vi "Get Response Fit.vi"(8 "error in (no error)":errorcluster, 11 "Exponential Fit in":refnum<class "Exponential Fit.lvclass">) -> (0 "error out":errorcluster, 2 "Fit out":dbl[](array[numeric]), 3 "Exponential Fit out":refnum<class "Exponential Fit.lvclass">)   [LabVIEW 2016, in "Exponential Fit.lvclass"]
uses:
  Exponential Fit.lvclass
  Exponential Fit.lvclass/Exponential Fit.ctl
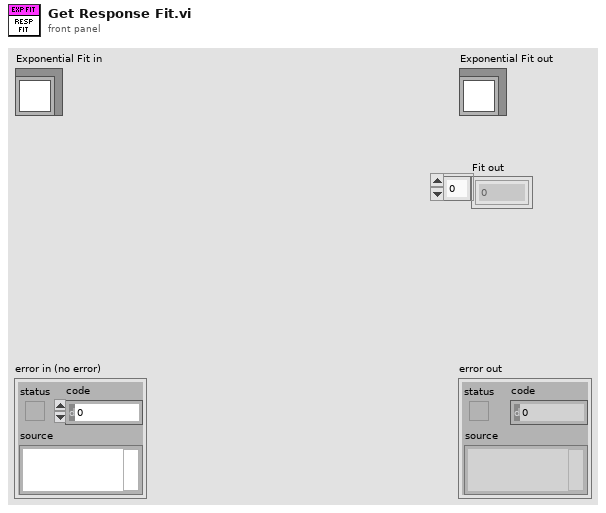
[diagram p1: front panel]
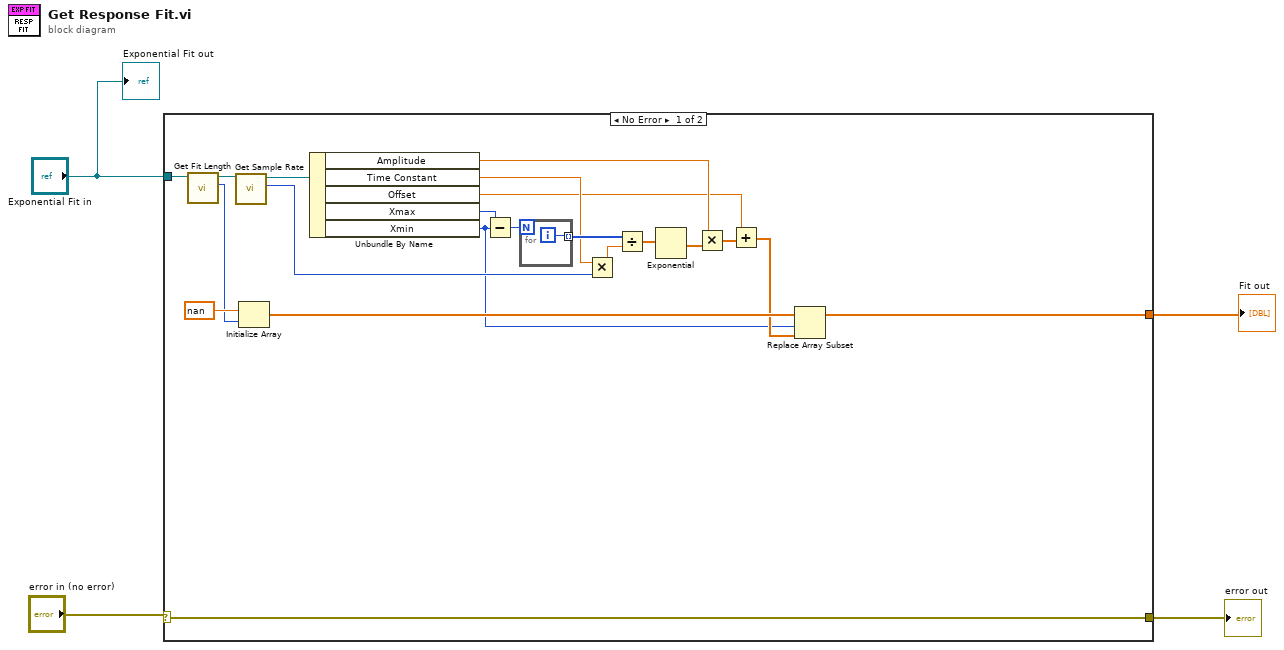
[diagram p0: block diagram]
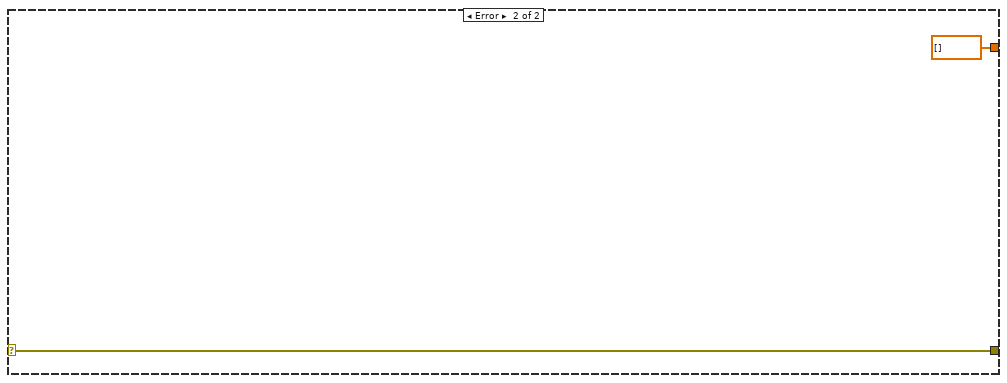
[diagram p2: hidden frame]
diagram:
  n1 = case shown="No Error" "error in (no error)" {
    selector: "error in (no error)" -> [w25 w28]
    tunnel: [w25 w28] -> w3
    tunnel: "Exponential Fit in" -> [w22 _]
    tunnel: [w5 dbl[] []] -> w1
    frame No Error {
      n2 = call-dynamic "Get Fit Length.vi"("Abstract Fit in"=w22) -> ("Length"=w9:i32, "Abstract Fit out"=w21:refnum<class "Exponential Fit.lvclass">)  [unwired: 8 in, 1 out]
      n3 = call-dynamic "Get Sample Rate.vi"("Abstract Fit in"=w21) -> ("Sample Rate"=w16:i32, "Abstract Fit out"=w20:refnum<class "Exponential Fit.lvclass">)  [unwired: 8 in, 1 out]
      n4 = Initialize Array(nan ("element"), w9) -> (w8:dbl[])
      n5 = Unbundle By Name(w20) -> ("Amplitude"=w14:dbl, "Time Constant"=w17:dbl, "Offset"=w11:dbl, "Xmax"=w24:i32, "Xmin"=w6:i32)
      n6 = Subtract(x=w24, y=w6) -> (x-y=w23:i32)
      n7 = for {
        N: w23 -> [_]
        tunnel: [w26] -> w19 mode=indexing
        i -> [w26]
      }
      n8 = Multiply(x=w17, y=w16) -> (x*y=w18:dbl)
      n9 = Divide(x=w19, y=w18) -> (x/y=w15:dbl[])
      n10 = Exponential(1:w15) -> (0:w13:dbl[])
      n11 = Multiply(x=w14, y=w13) -> (x*y=w12:dbl[])
      n12 = Add(x=w11, y=w12) -> (x+y=w7:dbl[])
      n13 = Replace Array Subset(array=w8, new element=w7, index=w6) -> (w5:dbl[])
    }
    frame Error {
    }
  }
  "error out" <- w3
  "Fit out" <- w1
  "Exponential Fit out" <- "Exponential Fit in"
